vi "MagnetControl_v2.vi"() -> ()   [LabVIEW 2014]
uses:
  <vilib>/MakerHub/LINX/Private/Local IO/LinxI2cWrite.vi
  <vilib>/MakerHub/LINX/Public/Utilities/Check Channel.vi
  <vilib>/MakerHub/LINX/Public/Utilities/Open Serial.vi
  <vilib>/MakerHub/LINX/Private/Utilties/Generate Error.vi
  <vilib>/MakerHub/LINX/LMH-LINX.lvlib
panel:
  out "Waveform Chart":sgl(graph)
  out "Magnetic Field (Oe)":dbl
  out "DAC Voltage":dbl(knob) scale=0.0..5.0
  out "DAC Output":u16
  out "Device Name":string
  out "Error Out":errorcluster
  in  "millisecond multiple":u32
  in  "stop":bool
  in  "DAC Output Voltage":sgl min=0 max=5 step=0.001
  in  "Serial Port":refnum<visa-resource-name>="N/A"
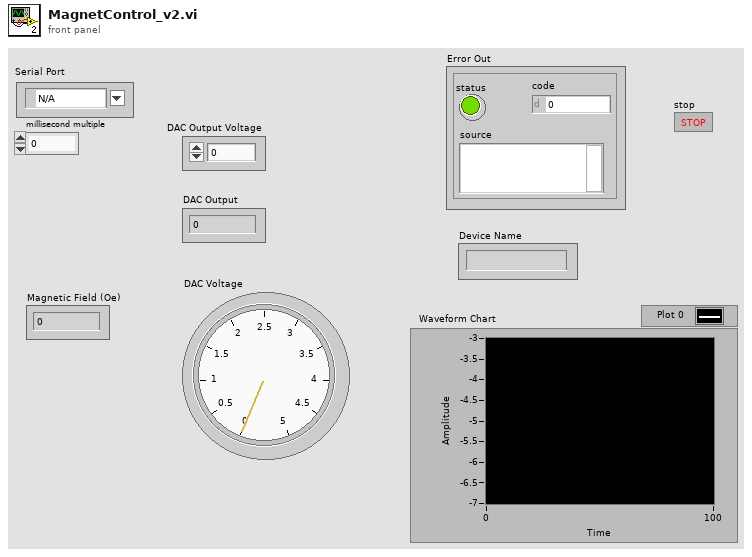
[diagram p1: front panel]
types:
  T1 = typedef "LMH-LINX.lvlib/LINX Ref.ctl" = cluster{"IO":T2, "Interface":T3, "LINX Device Config":T4}
  T2 = typedef "LMH-LINX.lvlib/Platform.ctl" = enum16{"Remote", "Local"}
  T3 = typedef "LMH-LINX.lvlib/Interface.ctl" = enum16{"Serial", "TCP"}
  T4 = typedef "LMH-LINX.lvlib/Device.lvlib/LINX Device Config.ctl" = cluster{"Interface":T3, "COM Port":refnum<visa-resource-name>, "TCP Configuration":T5, "Device Family":u8, "Device ID":u8, "Device Name":string, "TCP Ref":refnum<k5>, "Channels":T6}
  T5 = typedef "LMH-LINX.lvlib/Device.lvlib/TCP Config.ctl" = cluster{"IP Address":string, "Port":u16}
  T6 = typedef "LMH-LINX.lvlib/Channels.ctl" = cluster{"DI":u8[], "DO":u8[], "AI":u8[], "AO":u8[], "PWM":u8[], "QE":u8[], "UART":u8[], "I2C 2":u8[], "SPI":u8[], "CAN":u8[], "Servo":u8[], "AI Ref (V)":dbl, "AI Resolution (Bits)":u8, "AO Ref (V)":dbl, "AO Resolution (Bits)":u8}
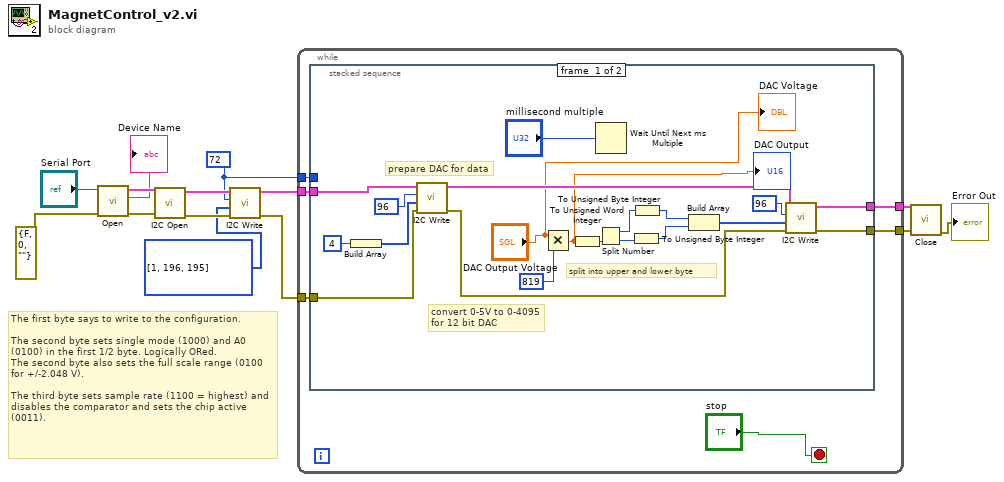
[diagram p0: block diagram]
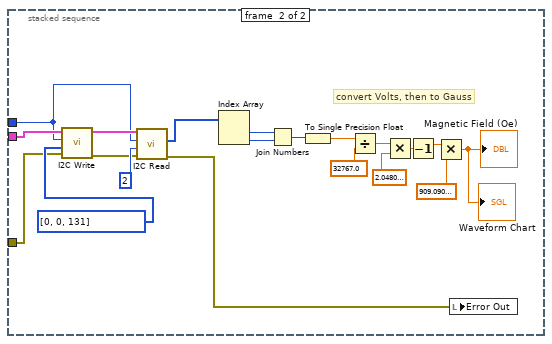
[diagram p2: hidden frame]
diagram:
  w1 = u8 72 ("I2C Slave Address (0)")
  # "The first byte says to write to the configuration.\n\nThe second byte sets single mode (1000) and A0 (0100) in the first 1/2 byte. Logically ORed.\nThe second byte also sets the full scale range (0100 for +/-2.048 V).\n\nThe third byte sets sample rate (1100 = highest) and disables the comparator and sets the chip active (0011)."
  n1 = call-poly <vilib>:"Open.vi"("Error In"=errorcluster {"status"=FALSE, "code"=0, "source"=""}, "Serial Port"="Serial Port") -> ("Error Out"=w12:errorcluster, "Device Name"=→"Device Name":string, "LINX Resource"=w13:T1)  [unwired: 7 in]
  n2 = call <vilib>:"I2C Open.vi"("Error In"=w12, "LINX Resource"=w13) -> ("Error Out"=w4:errorcluster, "LINX Resource"=w6:T1)  [unwired: 8 in]
  n3 = call <vilib>:"I2C Write.vi"("Error In"=w4, "Data"=u8[] [1, 196, 195], "I2C Slave Address (0)"=w1, "LINX Resource"=w6) -> ("Error Out"=w3:errorcluster, "LINX Resource"=w5:T1)  [unwired: 6 in]
  n4 = while {
    tunnel: w5 -> [w18]
    tunnel: w3 -> [w16]
    tunnel: [w20] -> w8
    tunnel: [w19] -> w7
    tunnel: w1 -> [w15]
    stop <- "stop" stop-if-true
    n5 = stacked-sequence {
      tunnel: [w40 _] -> w20
      tunnel: [w39 _] -> w19
      tunnel: w18 -> [w38 w43]
      tunnel: w16 -> [w37 w41]
      tunnel: w15 -> [_ w42]
      frame #0 {
        # "prepare DAC for data"
        # "convert 0-5V to 0-4095\nfor 12 bit DAC"
        # "split into upper and lower byte"
        n6 = Build Array(u8 4) -> (w22:u8[])
        n7 = call <vilib>:"I2C Write.vi"("Error In"=w37, "Data"=w22, "I2C Slave Address (0)"=u8 96, "LINX Resource"=w38) -> ("Error Out"=w26:errorcluster, "LINX Resource"=w25:T1)  [unwired: 6 in]
        n8 = Multiply(x="DAC Output Voltage", y=u32 819) -> (x*y=w24:sgl)
        "DAC Output" <- w24
        n9 = To Unsigned Word Integer(number=w24) -> (unsigned 16bit integer=w29:u16)
        n10 = Wait Until Next ms Multiple(millisecond multiple="millisecond multiple") -> ()  [unwired: 1 out]
        n11 = Split Number(x=w29) -> (hi(x)=w30:u8, lo(x)=w35:u8)
        n12 = To Unsigned Byte Integer(number=w35) -> (unsigned 8bit integer=w32:u8)
        n13 = To Unsigned Byte Integer(number=w30) -> (unsigned 8bit integer=w33:u8)
        n14 = Build Array(w33, w32) -> (w31:u8[])
        n15 = call <vilib>:"I2C Write.vi"("Error In"=w26, "Data"=w31, "I2C Slave Address (0)"=u8 96, "LINX Resource"=w25) -> ("Error Out"=w39:errorcluster, "LINX Resource"=w40:T1)  [unwired: 6 in]
        "DAC Voltage" <- "DAC Output Voltage"
      }
      frame #1 {
        # "convert Volts, then to Gauss"
        n16 = call <vilib>:"I2C Write.vi"("Error In"=w41, "Data"=u8[] [0, 0, 131], "I2C Slave Address (0)"=w42, "LINX Resource"=w43) -> ("Error Out"=w56:errorcluster, "LINX Resource"=w57:T1)  [unwired: 6 in]
        n17 = call <vilib>:"I2C Read.vi"("Error In"=w56, "Bytes To Read"=u8 2, "I2C Slave Address (0)"=w42, "LINX Resource"=w57) -> ("Error Out"=w44:errorcluster, "Data"=w59:u8[])  [unwired: 5 in, 1 out]
        n18 = Index Array(array=w59) -> (element #1=w53:u8, element #2=w52:u8)  [unwired: 2 in]
        n19 = Join Numbers(hi=w53, lo=w52) -> ((hi.lo)=w55:u16)
        n20 = To Single Precision Float(number=w55) -> (single precision float=w48:sgl)
        n21 = Divide(x=w48, y=sgl 32767.0) -> (x/y=w51:sgl)
        n22 = Multiply(x=w51, y=sgl 2.048) -> (x*y=w50:sgl)
        n23 = Decrement(x=w50) -> (x-1=w46:sgl)
        n24 = Multiply(x=w46, y=sgl 909.09) -> (x*y=→"Magnetic Field (Oe)" →"Waveform Chart":sgl)
        n25 = local write "Error Out"(w44) -> ()
      }
    }
  }
  n26 = call <vilib>:"Close.vi"("Error In"=w7, "LINX Resource"=w8) -> ("Error Out"=→"Error Out":errorcluster)  [unwired: 9 in]
